vi "test1.vi"() -> ()   [LabVIEW 2023]
uses:
  Interfaces/IConfigure/IConfigure.lvclass
  Interfaces/IRead Voltage/IRead Voltage.lvclass
  Voltmeter Virtual/Voltmeter Virtual.lvclass
panel:
  out "Voltage":dbl format="%#_g V"
  out "Error Out 2":errorcluster
  out "Error Out":errorcluster
  out "Waveform Chart":dbl(graph)
  in  "Stop":bool
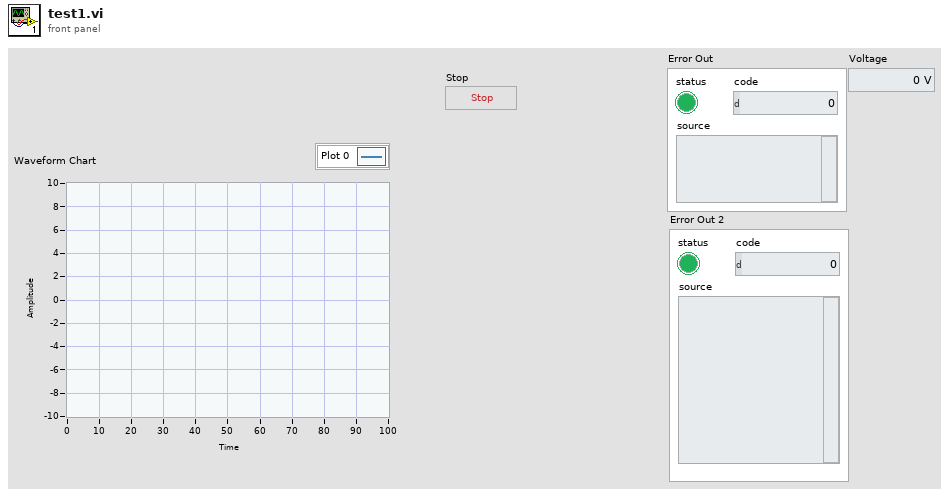
[diagram p1: front panel]
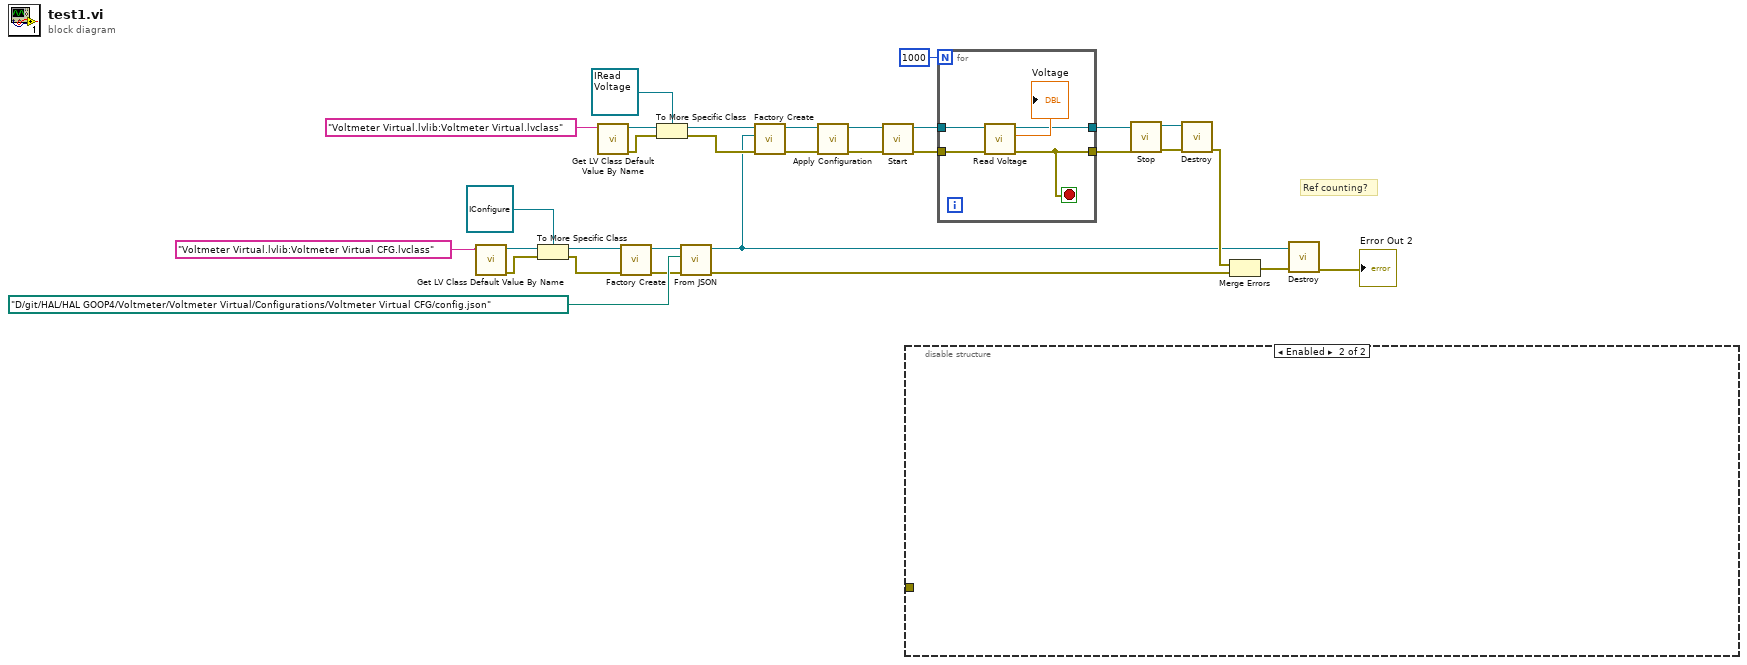
[diagram p0: block diagram]
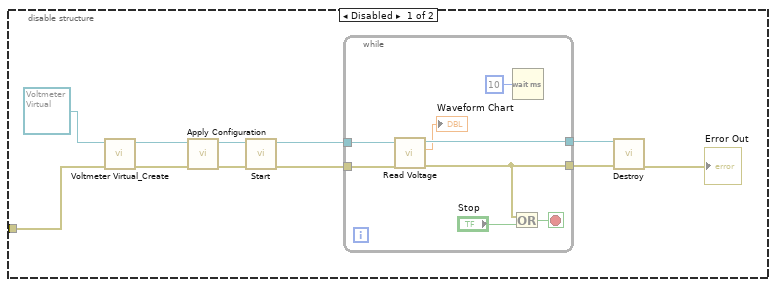
[diagram p2: hidden frame]
diagram:
  # "Ref counting?"
  n1 = call <vilib>:"Get LV Class Default Value By Name.vi"("class name"="Voltmeter Virtual.lvlib:Voltmeter Virtual CFG.lvclass") -> ("error out"=w25:errorcluster, "object"=w23:refnum<class>)  [unwired: 9 in]
  n2 = To More Specific Class(target class=refnum<class "IConfigure.lvclass"> refnum ("IConfigure"), reference=w23, error in=w25) -> (specific class reference=w26:refnum<class "IConfigure.lvclass">, error out=w24:errorcluster)
  n3 = call <vilib>:"Get LV Class Default Value By Name.vi"("class name"="Voltmeter Virtual.lvlib:Voltmeter Virtual.lvclass") -> ("error out"=w19:errorcluster, "object"=w21:refnum<class>)  [unwired: 9 in]
  n4 = call-dynamic "Factory Create.vi"("Error In"=w24, "object in"=w26) -> ("Error Out"=w29:errorcluster, "object out"=w31:refnum<class "IConfigure.lvclass">)  [unwired: 8 in]
  n5 = To More Specific Class(target class=refnum<class "IRead Voltage.lvclass"> refnum ("IRead Voltage"), reference=w21, error in=w19) -> (specific class reference=w18:refnum<class "IRead Voltage.lvclass">, error out=w17:errorcluster)
  n6 = call-dynamic "From JSON.vi"("Error In"=w29, "File Path"=path "D:/git/HAL/HAL GOOP4/Voltmeter/Voltmeter Virtual/Configurations/Voltmeter Virtual CFG/config.json", "object in"=w31) -> ("Error Out"=w4:errorcluster, "object out"=w3:refnum<class "IConfigure.lvclass">)  [unwired: 7 in]
  n7 = call-dynamic "Factory Create.vi"("Error In"=w17, "IConfigure"=w3, "object in"=w18) -> ("Error Out"=w15:errorcluster, "object out"=w16:refnum<class "IRead Voltage.lvclass">)  [unwired: 7 in]
  n8 = call-dynamic "Apply Configuration.vi"("Error In"=w15, "object in"=w16) -> ("Error Out"=w13:errorcluster, "object out"=w14:refnum<class "IRead Voltage.lvclass">)  [unwired: 8 in]
  n9 = call-dynamic "Start.vi"("Error In"=w13, "object in"=w14) -> ("Error Out"=w11:errorcluster, "object out"=w10:refnum<class "IRead Voltage.lvclass">)  [unwired: 8 in]
  n10 = disable-structure shown="Enabled" {
    disable-tunnel: _ -> [w42 _]
    frame Disabled {
      n11 = call "Voltmeter Virtual_Create.vi"("Error In"=w42, "reference in"=refnum<class "Voltmeter Virtual.lvclass"> refnum ("Voltmeter Virtual.lvlib:Voltmeter Virtual")) -> ("Error Out"=w33:errorcluster, "reference out"=w34:refnum<class "Voltmeter Virtual.lvclass">)  [unwired: 8 in]
      n12 = call-dynamic "Apply Configuration.vi"("Error In"=w33, "reference in"=w34) -> ("Error Out"=w40:errorcluster, "reference out"=w41:refnum<class "Voltmeter Virtual.lvclass">)  [unwired: 8 in]
      n13 = call-dynamic "Start.vi"("Error In"=w40, "reference in"=w41) -> ("Error Out"=w38:errorcluster, "reference out"=w39:refnum<class "Voltmeter Virtual.lvclass">)  [unwired: 8 in]
      n14 = while {
        tunnel: w39 -> [w50]
        tunnel: w38 -> [w49]
        tunnel: [w43] -> w36
        tunnel: [w47] -> w37
        stop <- w44 stop-if-true
        n15 = call-dynamic "Read Voltage.vi"("Error In"=w49, "reference in"=w50) -> ("Error Out"=w43:errorcluster, "Voltage"=→"Waveform Chart":dbl, "reference out"=w47:refnum<class "Voltmeter Virtual.lvclass">)  [unwired: 7 in]
        n16 = Or(x=w43, y="Stop") -> (x .or. y?=w44:bool)
        n17 = Wait (ms)(milliseconds to wait=u32 10) -> ()  [unwired: 1 out]
      }
      n18 = call-dynamic "Destroy.vi"("Error In"=w36, "reference in"=w37) -> ("Error Out"=→"Error Out":errorcluster)  [unwired: 8 in, 1 out]
    }
    frame Enabled {
    }
  }
  n19 = for {
    N: 1000 -> [_]
    tunnel: w11 -> [w55]
    tunnel: w10 -> [w54]
    tunnel: [w52] -> w9
    tunnel: [w51] -> w8
    stop <- w51 stop-if-true
    n20 = call-dynamic "Read Voltage.vi"("Error In"=w55, "object in"=w54) -> ("Error Out"=w51:errorcluster, "Voltage"=→"Voltage":dbl, "object out"=w52:refnum<class "IRead Voltage.lvclass">)  [unwired: 7 in]
  }
  n21 = call-dynamic "Stop.vi"("Error In"=w8, "object in"=w9) -> ("Error Out"=w6:errorcluster, "object out"=w7:refnum<class "IRead Voltage.lvclass">)  [unwired: 8 in]
  n22 = call-dynamic "Destroy.vi"("Error In"=w6, "object in"=w7) -> ("Error Out"=w5:errorcluster)  [unwired: 8 in, 1 out]
  n23 = Merge Errors(w5, w4) -> (w2:errorcluster)
  n24 = call-dynamic "Destroy.vi"("Error In"=w2, "object in"=w3) -> ("Error Out"=→"Error Out 2":errorcluster)  [unwired: 8 in, 1 out]
